vi "Received String to 2D Pixmap Array.vi"(8 "Width":i32, 9 "Height":i32, 11 "Receive Buffer":string) -> (3 "Array":u32[][](array[numeric]))   [LabVIEW 2025]
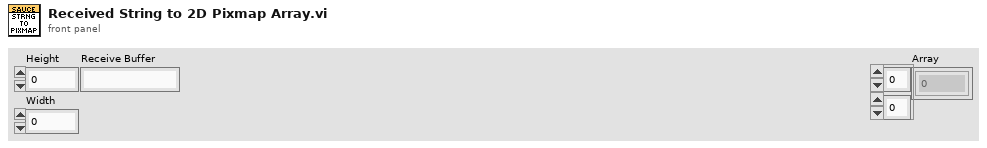
[diagram p1: front panel]
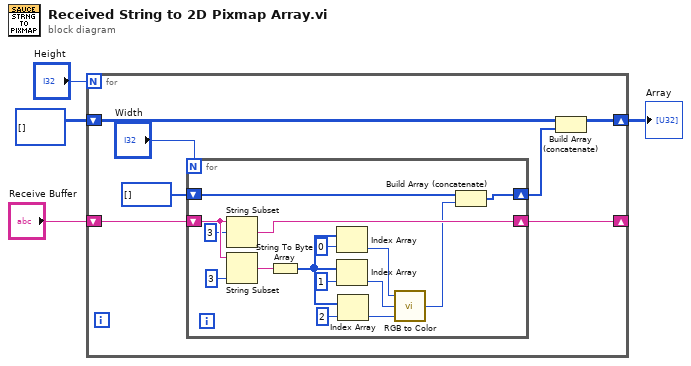
[diagram p0: block diagram]
diagram:
  n1 = for {
    N: "Height" -> [_]
    shift-right: [w11] -> _
    shift-left: "Receive Buffer" -> [w10]
    shift-right: [w6] -> w3
    shift-left: u32[][] [] -> [w8]
    n2 = for {
      N: "Width" -> [_]
      shift-right: [w26] -> w11
      shift-left: w10 -> [w16]
      shift-right: [w13] -> w7
      shift-left: u32[] [] -> [w14]
      n3 = String Subset(string=w16, offset (0)=3) -> (substring=w26:string)  [unwired: 1 in]
      n4 = String Subset(string=w16, length (rest)=3 ("length (rest)")) -> (substring=w24:string)  [unwired: 1 in]
      n5 = String To Byte Array(string=w24) -> (unsigned byte array=w23:u8[])
      n6 = Index Array(array=w23, index=0) -> (element=w18:u8)
      n7 = Index Array(array=w23, index=1) -> (element=w17:u8)
      n8 = Index Array(array=w23, index=2) -> (element=w19:u8)
      n9 = call <vilib>:"RGB to Color.vi"("B"=w19, "G"=w17, "R"=w18) -> ("Color"=w12:u32)
      n10 = Build Array (concatenate)(w14, w12) -> (w13:u32[])
    }
    n11 = Build Array (concatenate)(w8, w7) -> (w6:u32[][])
  }
  "Array" <- w3
